vi "Drive Calibration Processing.vi"(1 "Distance (Feet)":dbl format="%#_13g") -> (0 "Calibration Constant":dbl)   [LabVIEW 2013]
panel:
  out "Previous Values":dbl[](array[numeric])
  out "Last Run":dbl
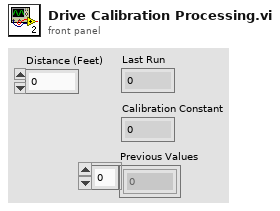
[diagram p1: front panel]
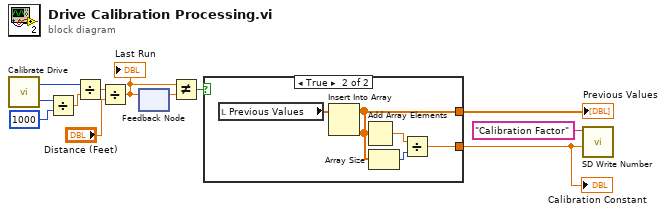
[diagram p0: block diagram]
diagram:
  n1 = call "Calibrate Drive.vi"() -> ("Time (ms)"=w11:u32, "Counts"=w12:i32)  [unwired: 2 in]
  n2 = Divide(x=w11, y=1000) -> (x/y=w10:dbl)
  n3 = Divide(x=w12, y=w10) -> (x/y=w8:dbl)
  n4 = Divide(x=w8, y="Distance (Feet)") -> (x/y=w5:dbl)
  "Last Run" <- w5
  n5 = feedback-in #1(w5) -> ()
  n6 = feedback #1() -> (w6:dbl)  [unwired: 1 in]
  n7 = Not Equal?(x=w5, y=w6) -> (x != y?=w4:bool)
  n8 = case shown="True" w4 {
    tunnel: [_ w14] -> w2
    tunnel: [_ w13] -> w3
    frame False {
    }
    frame True {
      n9 = local read "Previous Values"() -> (w17:dbl[])
      n10 = Insert Into Array(array=w17) -> (w13:dbl[])  [unwired: 2 in]
      n11 = Add Array Elements(numeric array=w13) -> (sum=w15:dbl)
      n12 = Array Size(array=w13) -> (size(s)=w16:i32)
      n13 = Divide(x=w15, y=w16) -> (x/y=w14:dbl)
    }
  }
  "Calibration Constant" <- w2
  "Previous Values" <- w3
  n14 = call <vilib>:"SD Write Number.vi"("Numeric"=w2, "Name"="Calibration Factor") -> ()  [unwired: 8 in, 2 out]
